vi "project1.vi"() -> ()   [LabVIEW 2021]
uses:
  <instrlib>/niDMM/nidmm.llb/niDMM Function.ctl
  <vilib>/express/express analysis/Spectral/Block/exnSpectralBlock spectral measurements RMS poly.vi
  <vilib>/express/express analysis/Spectral/XNode/ExpressSpectralMeasurementsBlockNode.xnode
  <vilib>/express/express analysis/Spectral/Block/exnSpectralBlock spectral measurements RMS DDT.vi
  <instrlib>/niSwitch/niSwitch.llb/niSwitch Connect Channels (Single).vi
  <instrlib>/niDMM/nidmm.llb/niDMM Configure Measurement Absolute.vi
panel:
  out "Spectral Analysis: Magnitude":dynamicdata(graph)
  in  "Number Of Drops":dbl
  in  "Path":path
  out "2nd Trigger":bool
  out "1st Trigger":bool
  out "Spectral Analysis: Phase":dynamicdata(graph)
  out "Time Series":dynamicdata(graph)
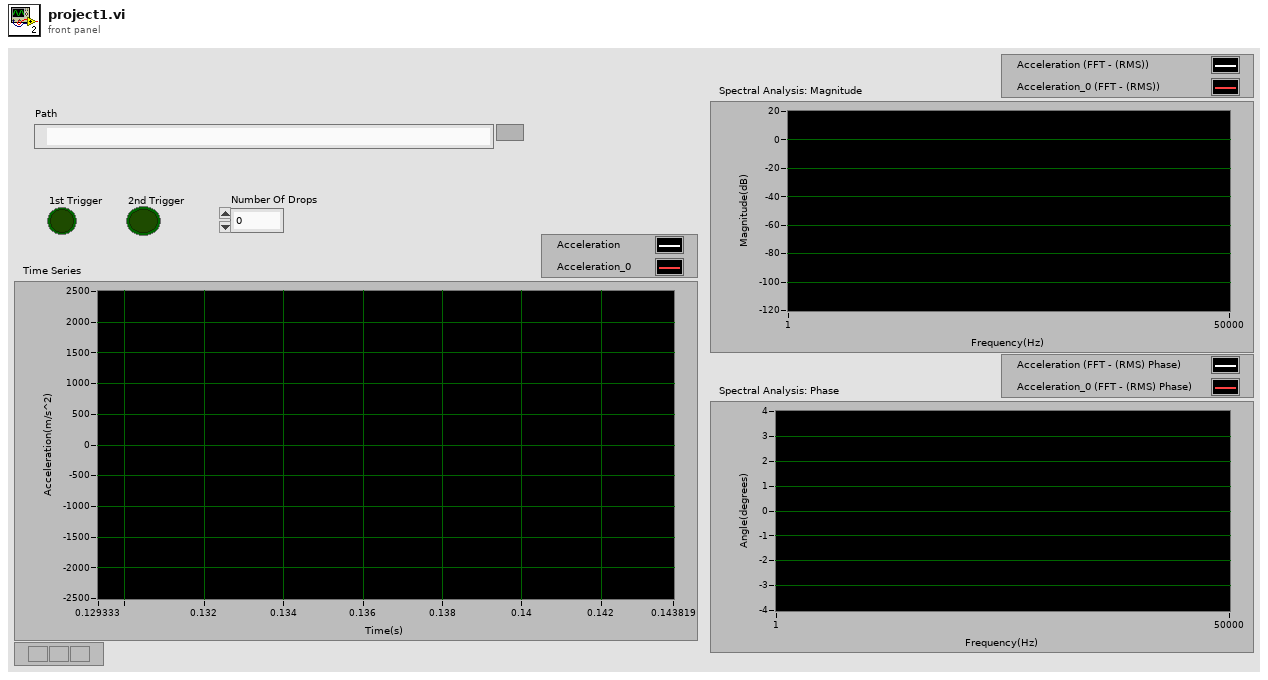
[diagram p1: front panel]
types:
  T1 = typedef "niDMM Function.ctl" = enum16{"DC Volts", "AC Volts", "DC Current", "AC Current", "2-wire Resistance", "4-wire Resistance", "Diode", "Frequency", "Period", "AC Volts DC Coupled", "Capacitance", "Inductance", "Temperature"}
  T2 = enum16{"open", "replace", "create", "open or create", "replace or create", "replace or create with confirmation"}
  T3 = cluster{"averaging mode":u16, "weighting mode":u16, "number of averages":u32}
  T4 = cluster{"dB On (F)":bool, "unwrap phase (F)":bool, "convert to degree (F)":bool}
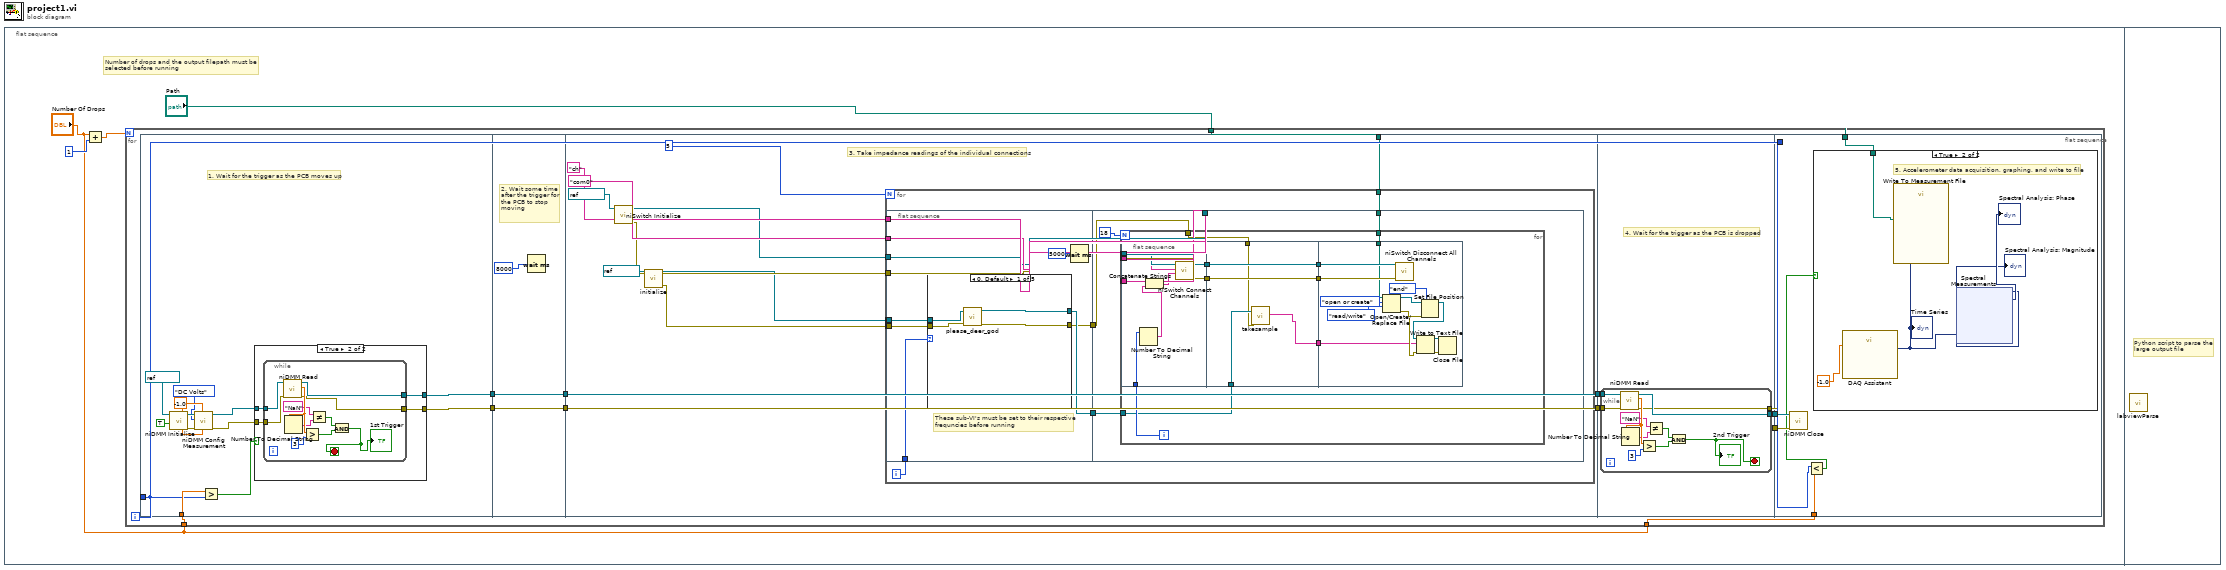
[diagram p0: block diagram]
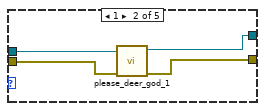
[diagram p3: hidden frame]
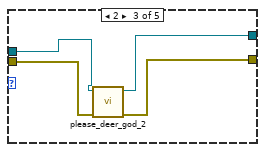
[diagram p4: hidden frame]
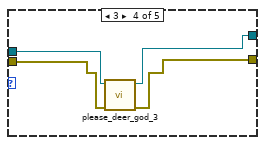
[diagram p5: hidden frame]
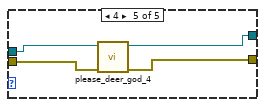
[diagram p6: hidden frame]
diagram:
  n1 = flat-sequence {
    frame #0 {
      # "Number of drops and the output filepath must be\nselected before running"
      n2 = Add(x="Number Of Drops", y=1) -> (x+y=w2:dbl)
      n3 = for {
        N: w2 -> [_]
        tunnel: "Path" -> [w12]
        tunnel: "Number Of Drops" -> [w11]
        tunnel: "Number Of Drops" -> [w10]
        i -> [w9]
        n4 = flat-sequence {
          tunnel: [w21] -> w8
          tunnel: [w20] -> w6
          tunnel: w10 -> [w19]
          tunnel: w9 -> [w18]
          tunnel: w8 -> [w49]
          tunnel: [w49] -> w7
          tunnel: w6 -> [w48]
          tunnel: [w48] -> w5
          tunnel: [w62] -> w16
          tunnel: w7 -> [w62]
          tunnel: [w61] -> w15
          tunnel: w5 -> [w61]
          tunnel: w12 -> [w50]
          tunnel: w16 -> [w149]
          tunnel: w15 -> [w148]
          tunnel: [w147] -> w14
          tunnel: [w146] -> w13
          tunnel: w14 -> [w166]
          tunnel: w13 -> [w165]
          tunnel: w12 -> [w164]
          tunnel: w9 -> [w163]
          tunnel: w11 -> [w162]
          frame #0 {
            w24 = -1.0
            # "1. Wait for the trigger as the PCB moves up"
            n5 = call <instrlib>:"niDMM Initialize.vi"("Reset"=TRUE, "Instrument Descriptor"=refnum<k15> "DMM") -> ("error out"=w26:errorcluster, "instrument handle out"=w27:refnum<k15>)  [unwired: 8 in]
            n6 = call-poly <instrlib>:"niDMM Config Measurement.vi"("Range"=w24, "Resolution"=w24, "error in (no error)"=w26, "Function"=niDMM_Function."DC Volts", "instrument handle"=w27) -> ("error out"=w29:errorcluster, "instrument handle out"=w28:refnum<k15>)  [unwired: 5 in]
            n7 = Greater?(x=w19, y=w18) -> (0:w17:bool)
            n8 = case shown="True" w17 {
              tunnel: w29 -> [w31 w35]
              tunnel: w28 -> [w30 w34]
              tunnel: [w30 w33] -> w21
              tunnel: [w31 w32] -> w20
              frame False {
              }
              frame True {
                n9 = while {
                  tunnel: w34 -> [w46]
                  tunnel: w35 -> [w45]
                  tunnel: [w38] -> w33
                  tunnel: [w37] -> w32
                  stop <- w36 stop-if-true
                  n10 = call <instrlib>:"niDMM Read.vi"("error in (no error)"=w45, "instrument handle"=w46) -> ("error out"=w37:errorcluster, "Measurement"=w43:dbl, "instrument handle out"=w38:refnum<k15>)  [unwired: 7 in]
                  n11 = Number To Decimal String(number=w43) -> (decimal integer string=w41:string)  [unwired: 1 in]
                  n12 = Greater?(x=w43, y=3) -> (0:w39:bool)
                  n13 = Not Equal?(x="NaN", y=w41) -> (x != y?=w40:bool)
                  n14 = And(x=w40, y=w39) -> (x .and. y?=w36:bool)
                  "1st Trigger" <- w36
                }
              }
            }
          }
          frame #1 {
            # "2. Wait some time\nafter the trigger for the PCB to stop moving"
            n15 = Wait (ms)(milliseconds to wait=u32 8000) -> ()  [unwired: 1 out]
          }
          frame #2 {
            # "3. Take impedance readings of the individual connections"
            n16 = call <instrlib>:"niSwitch Initialize.vi"("resource name"=refnum<k15> "switch") -> ("error out"=w55:errorcluster, "instrument handle out"=w54:refnum<k15>)  [unwired: 9 in]
            n17 = call "initialize.vi"("VISA resource name"=refnum<visa-resource-name> "COM7") -> ("error out"=w51:errorcluster, "VISA resource name out"=w52:refnum<visa-resource-name>)  [unwired: 8 in, 1 out]
            n18 = for {
              N: 5 -> [_]
              tunnel: "ch" -> [w72]
              tunnel: "com0" -> [w71]
              tunnel: w55 -> [w70]
              tunnel: w54 -> [w69]
              tunnel: w52 -> [w67]
              tunnel: w51 -> [w66]
              tunnel: w50 -> [w63]
              i -> [w68]
              n19 = flat-sequence {
                tunnel: w68 -> [w77]
                tunnel: w67 -> [w76]
                tunnel: w66 -> [w75]
                tunnel: [w74] -> w65
                tunnel: [w73] -> w64
                tunnel: w72 -> [w105]
                tunnel: w71 -> [w104]
                tunnel: w70 -> [w103]
                tunnel: w69 -> [w102]
                tunnel: w65 -> [w100]
                tunnel: w64 -> [w99]
                tunnel: w63 -> [w98]
                frame #0 {
                  # "These sub-VI's must be set to their respective\nfrequncies before running"
                  n20 = case shown="0, Default" w77 {
                    tunnel: w76 -> [w81 w85 w89 w93 w97]
                    tunnel: w75 -> [w80 w84 w88 w92 w94]
                    tunnel: [w79 w83 w86 w90 w96] -> w74
                    tunnel: [w78 w82 w87 w91 w95] -> w73
                    frame 0, Default {
                      n21 = call "please_deer_god.vi"("error out 2"=w80, "VISA resource name out"=w81) -> ("error out"=w78:errorcluster, "VISA resource name out 2"=w79:refnum<visa-resource-name>)  [unwired: 5 in]
                    }
                    frame 1 {
                      n22 = call "please_deer_god_1.vi"("error out 2"=w84, "VISA resource name out"=w85) -> ("error out"=w82:errorcluster, "VISA resource name out 2"=w83:refnum<visa-resource-name>)  [unwired: 8 in]
                    }
                    frame 2 {
                      n23 = call "please_deer_god_2.vi"("VISA resource name out"=w89, "error out 2"=w88) -> ("VISA resource name out 2"=w86:refnum<visa-resource-name>, "error out"=w87:errorcluster)  [unwired: 7 in]
                    }
                    frame 3 {
                      n24 = call "please_deer_god_3.vi"("VISA resource name out"=w93, "error out 2"=w92) -> ("VISA resource name out 2"=w90:refnum<visa-resource-name>, "error out"=w91:errorcluster)  [unwired: 6 in]
                    }
                    frame 4 {
                      n25 = call "please_deer_god_4.vi"("error out 2"=w94, "VISA resource name out"=w97) -> ("error out"=w95:errorcluster, "VISA resource name out 2"=w96:refnum<visa-resource-name>)  [unwired: 8 in]
                    }
                  }
                }
                frame #1 {
                  n26 = for {
                    N: 18 -> [_]
                    tunnel: w105 -> [w113]
                    tunnel: w104 -> [w112]
                    tunnel: w103 -> [w111]
                    tunnel: w102 -> [w110]
                    tunnel: w100 -> [w109]
                    tunnel: w99 -> [w108]
                    tunnel: w98 -> [w106]
                    i -> [w114]
                    n27 = flat-sequence {
                      tunnel: w110 -> [w127]
                      tunnel: w111 -> [w126]
                      tunnel: w112 -> [w125]
                      tunnel: [w124] -> w117
                      tunnel: [w123] -> w115
                      tunnel: w114 -> [w122]
                      tunnel: w113 -> [w119]
                      tunnel: [w132] -> w118
                      tunnel: w117 -> [w132]
                      tunnel: [w131] -> w116
                      tunnel: w115 -> [w131]
                      tunnel: w109 -> [w130]
                      tunnel: w108 -> [w129]
                      tunnel: [w128] -> w107
                      tunnel: w118 -> [w145]
                      tunnel: w116 -> [w144]
                      tunnel: w107 -> [w139]
                      tunnel: w106 -> [w137]
                      frame #0 {
                        n28 = Number To Decimal String(number=w122) -> (decimal integer string=w120:string)  [unwired: 1 in]
                        n29 = Concatenate Strings(w119, w120) -> (w121:string)
                        n30 = call-poly <instrlib>:"niSwitch Connect Channels.vi"("error in (no error)"=w126, "channel 2"=w121, "channel 1"=w125, "instrument handle"=w127) -> ("error out"=w123:errorcluster, "instrument handle out"=w124:refnum<k15>)  [unwired: 6 in]
                      }
                      frame #1 {
                        n31 = call "takesample.vi"("error in (no error)"=w129, "VISA resource name"=w130) -> ("current sample"=w128:string)  [unwired: 7 in, 2 out]
                      }
                      frame #2 {
                        n32 = Open/Create/Replace File(file path (use dialog)=w137, operation (0:open)=T2."open or create", access (0:read/write)=enum16{"read/write", "read-only", "write-only"}."read/write") -> (refnum out=w143:refnum<file>, error out=w142:errorcluster)  [unwired: 3 in, 1 out]
                        n33 = call <instrlib>:"niSwitch Disconnect All Channels.vi"("error in (no error)"=w144, "instrument handle"=w145) -> ()  [unwired: 8 in, 2 out]
                        n34 = Set File Position(refnum=w143, from (0:start)=enum16{"start", "end", "current"}."end", error in=w142) -> (refnum out=w141:refnum<file>, error out=w140:errorcluster)  [unwired: 1 in]
                        n35 = Write to Text File(file (use dialog)=w141, text=w139, error in=w140) -> (refnum out=w133:refnum<file>, error out=w134:errorcluster)  [unwired: 1 in, 1 out]
                        n36 = Close File(refnum=w133, error in=w134) -> ()  [unwired: 2 out]
                      }
                    }
                  }
                }
              }
            }
            n37 = Wait (ms)(milliseconds to wait=u32 5000) -> ()  [unwired: 1 out]
          }
          frame #3 {
            # "4. Wait for the trigger as the PCB is dropped"
            n38 = while {
              tunnel: w149 -> [w154]
              tunnel: w148 -> [w153]
              tunnel: [w152] -> w147
              tunnel: [w151] -> w146
              stop <- w150 stop-if-true
              n39 = call <instrlib>:"niDMM Read.vi"("error in (no error)"=w153, "instrument handle"=w154) -> ("error out"=w151:errorcluster, "Measurement"=w159:dbl, "instrument handle out"=w152:refnum<k15>)  [unwired: 7 in]
              n40 = Number To Decimal String(number=w159) -> (decimal integer string=w157:string)  [unwired: 1 in]
              n41 = Greater?(x=w159, y=3) -> (0:w155:bool)
              n42 = Not Equal?(x="NaN", y=w157) -> (x != y?=w156:bool)
              n43 = And(x=w156, y=w155) -> (x .and. y?=w150:bool)
              "2nd Trigger" <- w150
            }
          }
          frame #4 {
            n44 = call <instrlib>:"niDMM Close.vi"("error in (no error)"=w165, "instrument handle"=w166) -> ()  [unwired: 9 in, 1 out]
            n45 = Less?(x=w163, y=w162) -> (x < y?=w161:bool)
            n46 = case shown="True" w161 {
              tunnel: w164 -> [_ w169]
              frame False {
              }
              frame True {
                # "5. Accelerometer data acquisition, graphing, and write to file"
                n47 = call "DAQ Assistant"("timeout (s)"=-1.0) -> ("data"=w170:dynamicdata)  [unwired: 16 in, 2 out]
                "Time Series" <- w170
                n48 = call "Write To Measurement File"("Signals"=w170, "Filename"=w169) -> ()  [unwired: 15 in, 3 out]
                n49 = xnode "Spectral Measurements"("Signals"=w170) -> ("FFT - (RMS)"=→"Spectral Analysis: Magnitude":dynamicdata, "Phase"=→"Spectral Analysis: Phase":dynamicdata)  [unwired: 1 in, 1 out]
              }
            }
          }
        }
      }
    }
    frame #1 {
      # "Python script to parse the\nlarge output file"
      n50 = call "labviewParse.vi"() -> ()  [unwired: 12 in]
    }
  }
